vi "Read Temperature (Raw).vi"(8 "error in (no error)":errorcluster, 11 "LPS Barometer in":refnum<class "LPS Barometric Pressure Sensor.lvclass">) -> (0 "error out":errorcluster, 2 "Raw Temperature":i16, 3 "LPS Barometer out":refnum<class "LPS Barometric Pressure Sensor.lvclass">)   [LabVIEW 2020, in "LPS Barometric Pressure Sensor.lvclass"]
doc: "Reads the raw temperature value from the device."
uses:
  LPS Barometric Pressure Sensor.lvclass
  LINX I2C/LINX I2C.lvclass
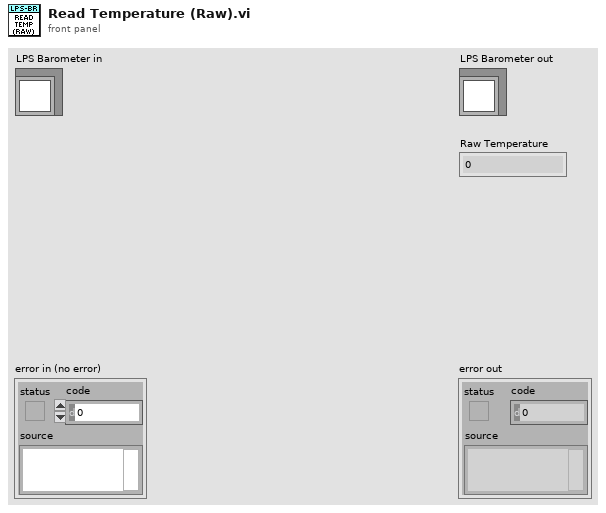
[diagram p1: front panel]
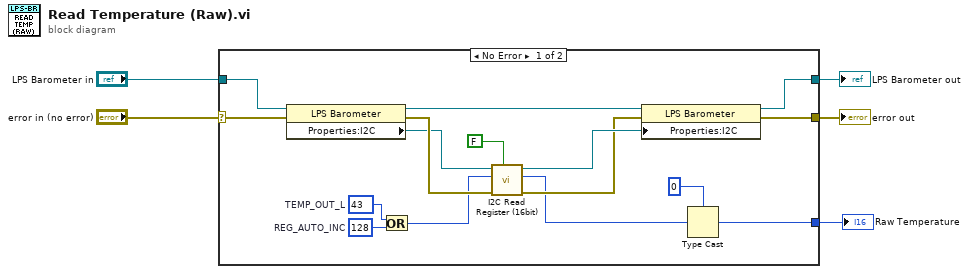
[diagram p0: block diagram]
diagram:
  n1 = case shown="No Error" "error in (no error)" {
    selector: "error in (no error)" -> [w18 w23]
    tunnel: [w17 w23] -> w4
    tunnel: [w19 w22] -> w2
    tunnel: "LPS Barometer in" -> [w21 w22]
    tunnel: [w13 _] -> w1
    frame No Error {
      w15 = u8 128  # REG_AUTO_INC
      w16 = u8 43  # TEMP_OUT_L
      n2 = property class="LPS Barometer"(reference=w21, error in=w18) -> (reference out=w20:refnum<class "LPS Barometric Pressure Sensor.lvclass">, error out=w12:errorcluster, "Properties:I2C"=w11:refnum<class "LINX I2C.lvclass">)
      n3 = Or(x=w16, y=w15) -> (x .or. y?=w7:u8)
      n4 = call "I2C Read Register (16bit).vi"("MSB(yte) First? (F=Lo->Hi)"=FALSE, "error in (no error)"=w12, "Register Address"=w7, "LINX I2C in"=w11) -> ("error out"=w9:errorcluster, "Value"=w8:u16, "LINX I2C out"=w10:refnum<class "LINX I2C.lvclass">)  [unwired: 5 in]
      n5 = property class="LPS Barometer"(reference=w20, error in=w9, "Properties:I2C"=w10) -> (reference out=w19:refnum<class "LPS Barometric Pressure Sensor.lvclass">, error out=w17:errorcluster)
      n6 = Type Cast(type=i16 0, x=w8) -> (*(type *) &x=w13:i16)
    }
    frame Error {
    }
  }
  "error out" <- w4
  "LPS Barometer out" <- w2
  "Raw Temperature" <- w1
